vi "S2C_CustomError.vi"(8 "Error In":errorcluster, 10 "Addiitional Info":string, 11 "Code":i32) -> (0 "Error Out":errorcluster)   [LabVIEW 2015]
doc: "Performs a lookup of the custom error code and appends any additional information to the error."
uses:
  <vilib>/Utility/error.llb/DialogType.ctl
  Globals/S2C_Globals.vi
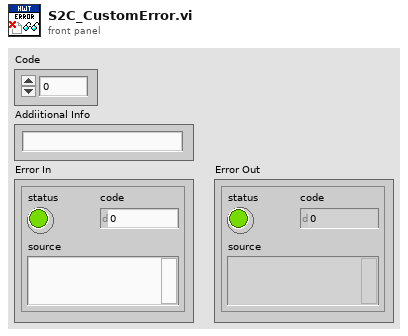
[diagram p1: front panel]
types:
  T1 = typedef "DialogType.ctl" = u16
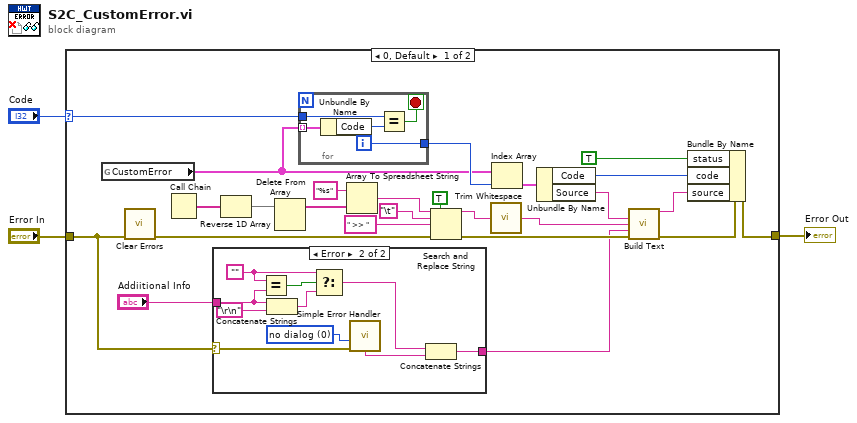
[diagram p0: block diagram]
diagram:
  n1 = case shown="0, Default" "Code" {
    selector: "Code" -> [w27 _]
    tunnel: "Error In" -> [w6 w45]
    tunnel: [w12 w45] -> w1
    frame 0, Default {
      n2 = global read "S2C_Globals.vi" "CustomError"() -> (w5:cluster{"Code":i32, "Source":string}[])
      n3 = call <vilib>:"Clear Errors.vi"("error in (no error)"=w6) -> ("error out"=w11:errorcluster)  [unwired: 5 in, 1 out]
      n4 = Call Chain() -> (call chain=w18:string[])
      n5 = case shown="Error" w6 {
        selector: w6 -> [_ w34]
        tunnel: [w29 w30] -> w10
        tunnel: "Addiitional Info" -> [w29 w37]
        frame No Error {
        }
        frame Error {
          w33 = T1 0 items=["no dialog", "OK message", "continue or stop message", "OK message + warnings", "continue/stop + warnings"] ("type of dialog (OK msg:1)")
          w35 = ""
          n6 = Equal?(x=w35, y=w37) -> (x = y?=w39:bool)
          n7 = Concatenate Strings(w37, "\r\n") -> (w38:string)
          n8 = Select(t=w35, s=w39, f=w38) -> (s? t:f=w32:string)
          n9 = call <vilib>:"Simple Error Handler.vi"("type of dialog (OK msg:1)"=w33, "error in (no error)"=w34) -> ("message"=w31:string)  [unwired: 3 in, 4 out]
          n10 = Concatenate Strings(w32, w31) -> (w30:string)
        }
      }
      n11 = Reverse 1D Array(array=w18) -> (reversed array=w17:string[])
      n12 = Delete From Array(array=w17) -> (array with subset deleted=w16:string[])  [unwired: 2 in, 1 out]
      n13 = for {
        tunnel: w5 -> [w44] mode=indexing
        tunnel: w27 -> [w41]
        tunnel: [w40] -> w26
        i -> [w40]
        stop <- w42 stop-if-true
        n14 = Unbundle By Name(w44) -> ("Code"=w43:i32)
        n15 = Equal?(x=w41, y=w43) -> (x = y?=w42:bool)
      }
      n16 = Array To Spreadsheet String(array=w16, 3:"%s" ("format string")) -> (spreadsheet string=w22:string)  [unwired: 1 in]
      n17 = Search and Replace String(replace all?=TRUE ("replace all? (F)"), input string=w22, search string="\t", replace string=" >> ", error in=w11) -> (result string=w15:string, error out=w23:errorcluster)  [unwired: 3 in, 2 out]
      n18 = call <vilib>:"Trim Whitespace.vi"("string"=w15) -> ("trimmed string"=w7:string)  [unwired: 1 in]
      n19 = Index Array(array=w5, index=w26) -> (element=w28:cluster{"Code":i32, "Source":string})
      n20 = Unbundle By Name(w28) -> ("Code"=w13:i32, "Source"=w8:string)
      n21 = call "Build Text"("Msg"=w8, "Source"=w7, "Info"=w10, "error in (no error)"=w23) -> ("Result"=w9:string, "error out"=w14:errorcluster)  [unwired: 10 in]
      n22 = Bundle By Name(cluster=w14, "status"=TRUE, "code"=w13, "source"=w9) -> (w12:errorcluster)
    }
    frame -1 {
    }
  }
  "Error Out" <- w1
